vi "Read Count Measurement (Serial Bus - CAN).vi"(8 "error in (no error)":errorcluster, 10 "Serial Bus Name (1: Serial Bus 1)":i32(ring)=1 items=["Serial Bus 1"=1, "Serial Bus 2"=2], 11 "VISA resource name":refnum<visa-resource-name>) -> (0 "error out":errorcluster, 1 "Overload Frame Count":dbl, 2 "Error Frame Count":dbl, 3 "VISA resource name out":refnum<visa-resource-name>, 4 "Utilization":dbl, 5 "Total Frame Count":dbl)   [LabVIEW 2010, in "Agilent 2000 3000 X-Series.lvlib"]
doc: "Returns the measurement of serial bus - CAN."
uses:
  <instrlib>/Agilent 2000 3000 X-Series/Agilent 2000 3000 X-Series.lvlib
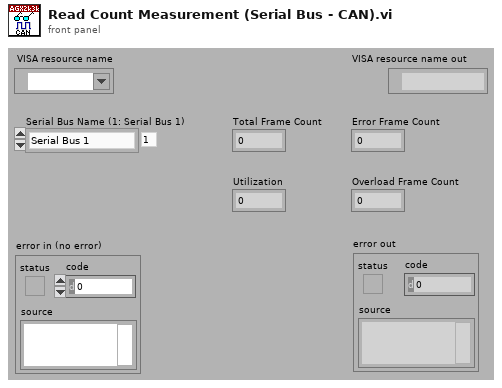
[diagram p1: front panel]
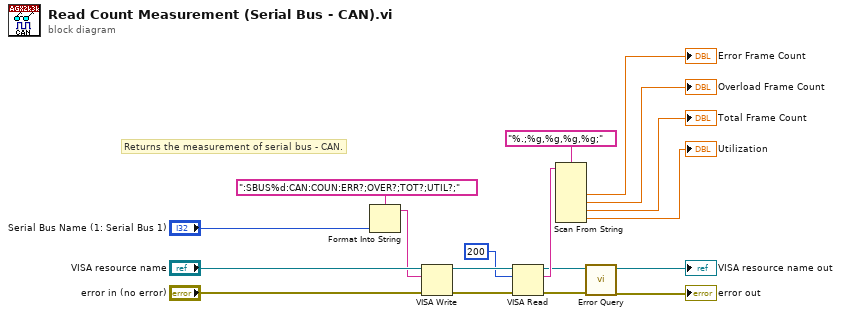
[diagram p0: block diagram]
diagram:
  # "Returns the measurement of serial bus - CAN."
  n1 = Format Into String(format string=":SBUS%d:CAN:COUN:ERR?;OVER?;TOT?;UTIL?;", "Serial Bus Name (1: Serial Bus 1)") -> (resulting string=w12:string)  [unwired: 2 in, 1 out]
  n2 = VISA Write(VISA resource name="VISA resource name", write buffer=w12, error in (no error)="error in (no error)") -> (VISA resource name out=w10:refnum<visa-resource-name>, error out=w9:errorcluster)  [unwired: 1 out]
  n3 = VISA Read(VISA resource name=w10, byte count=u32 200, error in (no error)=w9) -> (VISA resource name out=w8:refnum<visa-resource-name>, read buffer=w11:string, error out=w7:errorcluster)  [unwired: 1 out]
  n4 = Scan From String(format string="%.;%g,%g,%g,%g;", input string=w11) -> (output 1=→"Error Frame Count":dbl, output 2=→"Overload Frame Count":dbl, output 3=→"Total Frame Count":dbl, output 4=→"Utilization":dbl)  [unwired: 2 in, 7 out]
  n5 = call <instrlib>:"Error Query.vi"("error in (no error)"=w7, "VISA resource name"=w8) -> ("error out"=→"error out":errorcluster, "VISA resource name out"=→"VISA resource name out":refnum<visa-resource-name>)  [unwired: 8 out]
